vi "MeterPerSecond_To_RPM.vi"(4 "Wheel Radius (in meters)":dbl, 6 "Gearbox Reduction":dbl, 10 "m/s":dbl) -> (2 "RPM":dbl)   [LabVIEW 2019]
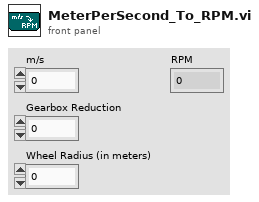
[diagram p1: front panel]
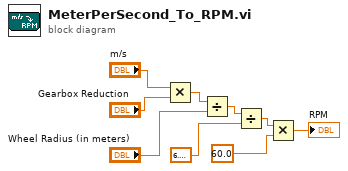
[diagram p0: block diagram]
diagram:
  n1 = Multiply(x="m/s", y="Gearbox Reduction") -> (x*y=w7:dbl)
  n2 = Divide(x=w7, y="Wheel Radius (in meters)") -> (x/y=w5:dbl)
  n3 = Divide(x=w5, y=6.283185307179586) -> (x/y=w3:dbl)
  n4 = Multiply(x=w3, y=60.0) -> (x*y=→"RPM":dbl)
